vi "Time to Day-Hr-Min-Sec-msec.vi"(2 "Time in millisec":dbl[](array[numeric]) format="%#.1f") -> (7 "Time Day/Hr:Min:Sec:msec":string[](array[string]))   [LabVIEW 2015, in "Powermeter_library.lvlib"]
doc: "Converts time in milliseconds to string Day/Hr:Min:Sec.msec"
uses:
  Powermeter_library.lvlib
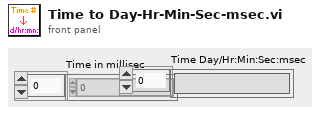
[diagram p1: front panel]
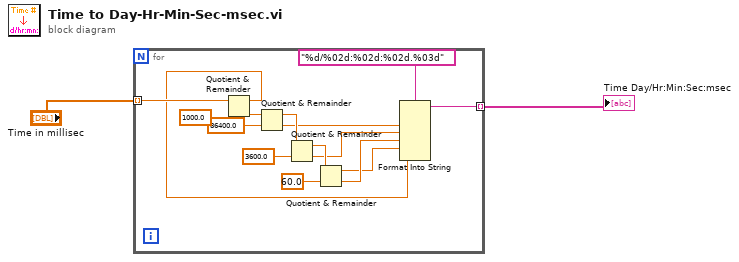
[diagram p0: block diagram]
diagram:
  n1 = for {
    tunnel: "Time in millisec" -> [w17] mode=indexing
    tunnel: [w3] -> w1 mode=indexing
    n2 = Quotient & Remainder(x=w17, y=1000.0) -> (x-y*floor(x/y)=w5:dbl, floor(x/y)=w15:dbl)
    n3 = Quotient & Remainder(x=w15, y=86400.0) -> (x-y*floor(x/y)=w13:dbl, floor(x/y)=w9:dbl)
    n4 = Quotient & Remainder(x=w13, y=3600.0) -> (x-y*floor(x/y)=w11:dbl, floor(x/y)=w8:dbl)
    n5 = Quotient & Remainder(x=w11, y=60.0) -> (x-y*floor(x/y)=w6:dbl, floor(x/y)=w7:dbl)
    n6 = Format Into String(format string="%d/%02d:%02d:%02d.%03d", w9, w8, w7, w6, w5) -> (resulting string=w3:string)  [unwired: 2 in, 1 out]
  }
  "Time Day/Hr:Min:Sec:msec" <- w1
